vi "Test_WriteString_NoFormatString_WriteExactString.vi"(8 "error in (no error)":errorcluster, 11 "TestBooleanTextBinding In":refnum<class "TestBooleanTextBinding.lvclass">) -> (0 "error out":errorcluster, 3 "TestBooleanTextBinding Out":refnum<class "TestBooleanTextBinding.lvclass">)   [LabVIEW 2017, in "TestBooleanTextBinding.lvclass"]
uses:
  TestBooleanTextBinding.lvclass
  Source/Concrete/BooleanTextBinding/BooleanTextBinding.lvclass/BooleanTextBinding.ctl
  Source/Concrete/BooleanTextBinding/BooleanTextBinding.lvclass
  C:/Git/composed-transport/Source/ITransport/ITransport.lvclass
  <vilib>/Utility/error.llb/Error Cluster From Error Code.vi
  Source/ITransport/ITransport.lvclass
panel:
  in  "OK Button":bool
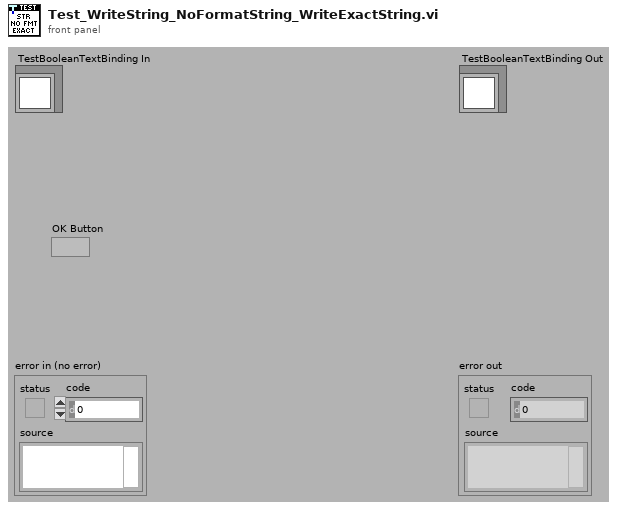
[diagram p1: front panel]
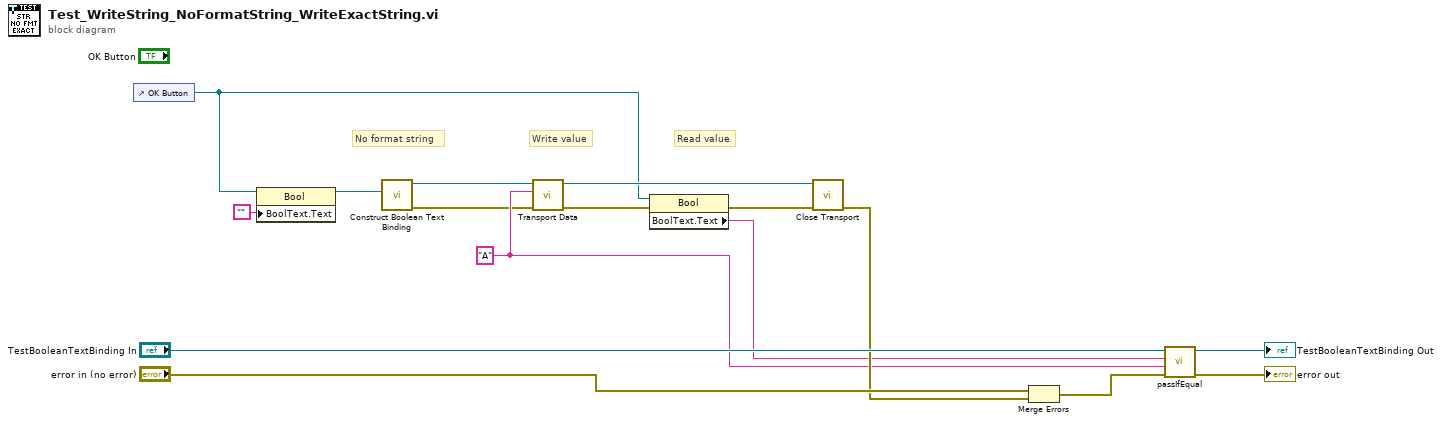
[diagram p0: block diagram]
diagram:
  w3 = "A" ("Format String")
  # "Read value"
  # "No format string"
  # "Write value"
  n1 = control-ref of="OK Button"() -> (w2:refnum<vi>)
  n2 = property class="Bool"(reference=w2, "BoolText.Text"="") -> (reference out=w8:refnum<vi>)  [unwired: 1 in, 1 out]
  n3 = call "Construct Boolean Text Binding.vi"("Bool Refnum"=w8) -> ("error out"=w1:errorcluster, "BooleanTextBinding"=w12:refnum<class "BooleanTextBinding.lvclass">)  [unwired: 9 in]
  n4 = call "Transport Data.vi"("error in (no error)"=w1, "Value"=w3, "ITransport in"=w12) -> ("error out"=w6:errorcluster, "ITransport out"=w10:refnum<class "BooleanTextBinding.lvclass">)  [unwired: 7 in]
  n5 = property class="Bool"(reference=w2, error in=w6) -> (error out=w5:errorcluster, "BoolText.Text"=w4:string)  [unwired: 1 out]
  n6 = call-dynamic "Close Transport.vi"("error in (no error)"=w5, "ITransport in"=w10) -> ("error out"=w9:errorcluster)  [unwired: 9 in]
  n7 = Merge Errors("error in (no error)", w9) -> (w11:errorcluster)
  n8 = call-dynamic "passIfEqual.vi"("error in (no error)"=w11, "y"=w3, "x"=w4, "TestCase in"="TestBooleanTextBinding In") -> ("error out"=→"error out":errorcluster, "TestCase out"=→"TestBooleanTextBinding Out":refnum<class "TestBooleanTextBinding.lvclass">)  [unwired: 6 in]
